vi "NewProductDialog.vi"(8 "error in (no error)":errorcluster, 11 "Product":T1) -> (0 "error out":errorcluster, 2 "Cancelled ?":bool, 3 "Product 2":T1)   [LabVIEW 2020]
doc: "Function generates data of new product."
uses:
  #typedef_Products.ctl
panel:
  in  "Cancel Button":bool
  in  "OK Button":bool
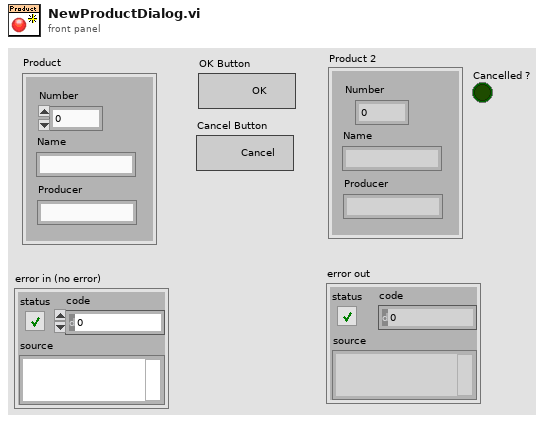
[diagram p1: front panel]
types:
  T1 = typedef "#typedef_Products.ctl" = cluster{"Number":dbl, "Name ":string, "Producer":string}
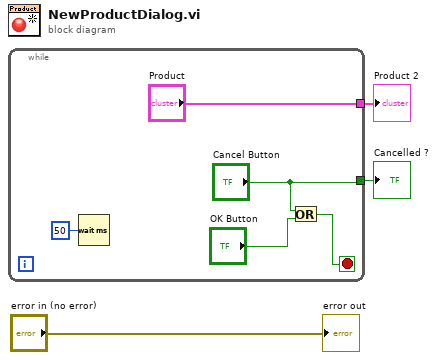
[diagram p0: block diagram]
diagram:
  n1 = while {
    tunnel: ["Product"] -> w3
    tunnel: ["Cancel Button"] -> w1
    stop <- w8 stop-if-true
    n2 = Wait (ms)(milliseconds to wait=u32 50) -> ()  [unwired: 1 out]
    n3 = Or(x="Cancel Button", y="OK Button") -> (x .or. y?=w8:bool)
  }
  "Product 2" <- w3
  "Cancelled ?" <- w1
  "error out" <- "error in (no error)"
